vi "Facade.vi"(0 "Data In":T5, 2 "Display State In":T2, 3 "Container State":T4) -> (6 "Data Out":T5, 7 "Display State Out":T2, 8 "Action":T1)   [LabVIEW 2013, in "BarCodes.lvlib" / "Barcode.xctl"]
uses:
  Barcode.xctl
  Data.ctl
  <vilib>/_xctls/Container State.ctl
  State.ctl
  BarcodeType.ctl
  <vilib>/_xctls/Action.ctl
  EAN-13/EAN-13.lvclass
  Code39/Code39.lvclass
  Code128/Code128.lvclass
  UPC/UPC.lvclass
  Linear Barcode/Linear Barcode.lvclass
  BarCode/Write Dark Color.vi
  BarCode/Write Light Color.vi
  BarCode/Write Scale.vi
  <vilib>/_xctls/XControlSupport.lvlib
  BarCodes.lvlib
panel:
  out "Barcode":picture
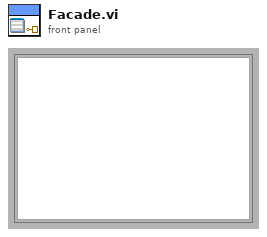
[diagram p1: front panel]
types:
  T1 = typedef "XControlSupport.lvlib/Action.ctl" = cluster{"Data Changed?":bool, "State Changed?":bool, "Action Name":string}
  T2 = typedef "BarCodes.lvlib/Barcode.xctl/State.ctl" = cluster{"BarcodeType":T3, "Scale":u8, "Dark Color":u32, "Light Color":u32}
  T3 = typedef "BarCodes.lvlib/BarcodeType.ctl" = enum16{"EAN-13", "UPC", "Code 39 (3 of 9)", "Code 128"}
  T4 = typedef "XControlSupport.lvlib/Container State.ctl" = cluster{"Indicator?":bool, "Run Mode?":bool, " Refnum":refnum<vi>}
  T5 = typedef "BarCodes.lvlib/Barcode.xctl/Data.ctl" = string
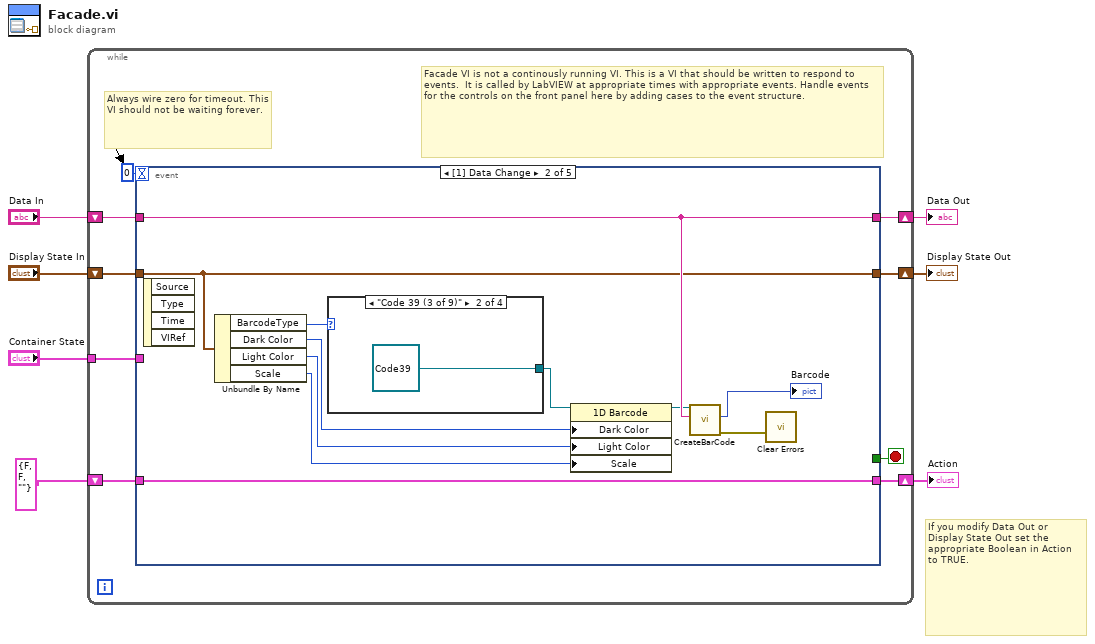
[diagram p0: block diagram]
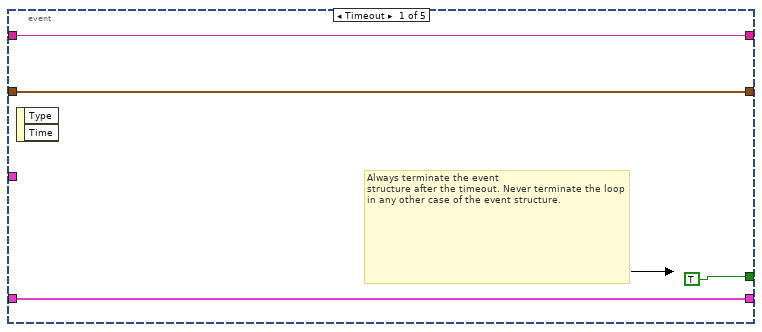
[diagram p2: hidden frame]
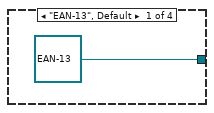
[diagram p3: hidden frame]
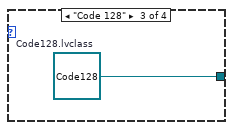
[diagram p4: hidden frame]
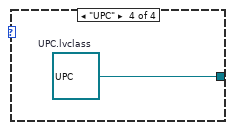
[diagram p5: hidden frame]
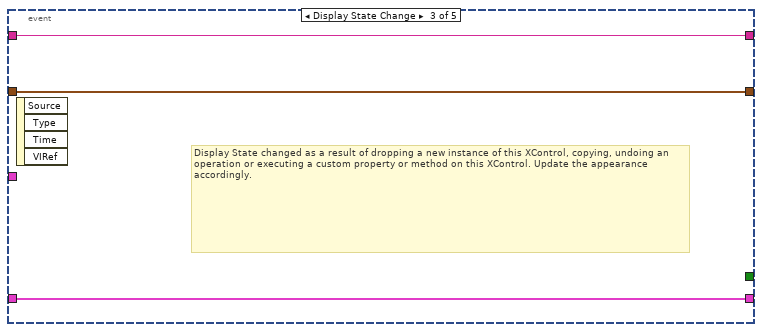
[diagram p6: hidden frame]
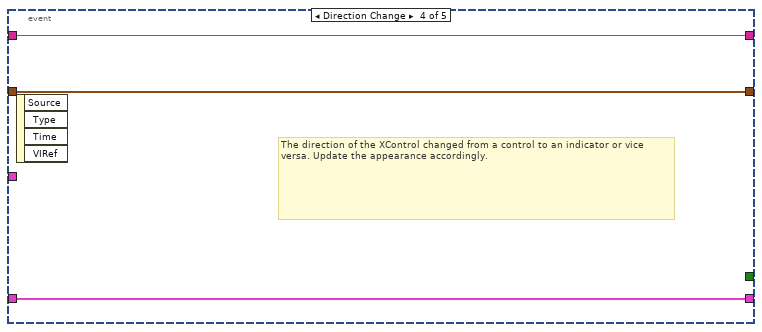
[diagram p7: hidden frame]
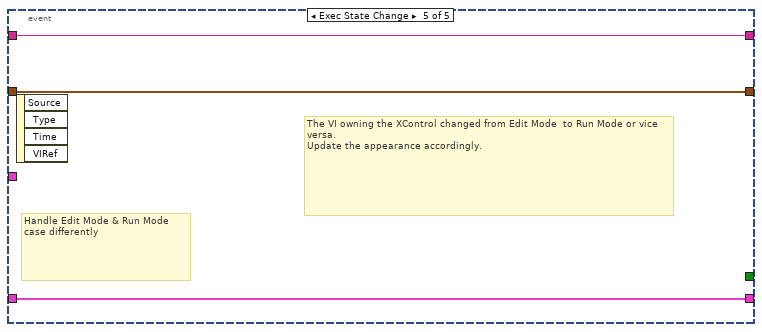
[diagram p8: hidden frame]
diagram:
  # "If you modify Data Out or\nDisplay State Out set the\nappropriate Boolean in Action\nto TRUE."
  n1 = while {
    shift-right: [w15] -> w4
    shift-left: "Display State In" -> [w16]
    tunnel: "Container State" -> [w12]
    shift-right: [w10] -> w7
    shift-left: "Data In" -> [w11]
    shift-right: [w8] -> w2
    shift-left: T1 {"Data Changed?"=FALSE, "State Changed?"=FALSE, "Action Name"=""} ("Action") -> [w9]
    stop <- w14 stop-if-true
    # "Facade VI is not a continously running VI. This is a VI that should be written to respond to events.  It is called by LabVIEW at appropriate times with appropriate events. Handle events for the controls on the front panel here by adding cases to the event structure."
    # "Always wire zero for timeout. This\nVI should not be waiting forever."
    n2 = event shown="[1] Data Change" {
      selector: _ -> [_ _ _ _ _]
      dyn-events: _ -> [_ _ _ _ _]
      timeout: 0 -> [_ _ _ _ _]
      tunnel: w16 -> [w18 w29 w38 w41 w44]
      tunnel: [w18 w29 w38 w41 w44] -> w15
      tunnel: [TRUE _ _ _ _] -> w14
      tunnel: w12 -> [_ _ _ _ _]
      tunnel: w11 -> [w17 w30 w37 w40 w43]
      tunnel: [w17 w30 w37 w40 w43] -> w10
      tunnel: [w19 w31 w36 w39 w42] -> w8
      tunnel: w9 -> [w19 w31 w36 w39 w42]
      event Timeout {
        # "Always terminate the event\nstructure after the timeout. Never terminate the loop in any other case of the event structure."
        n3 = event-data() -> ()  [unwired: 1 in, 2 out]
      }
      event Data Change {
        n4 = event-data() -> ()  [unwired: 1 in, 4 out]
        n5 = Unbundle By Name(w29) -> ("BarcodeType"=w28:T3, "Dark Color"=w24:u32, "Light Color"=w23:u32, "Scale"=w22:u8)
        n6 = case shown="\"Code 39 (3 of 9)\"" w28 {
          tunnel: [refnum<class "EAN-13.lvclass"> refnum ("EAN-13.lvclass") refnum<class "Code39.lvclass"> refnum ("Code39.lvclass") w34 w35] -> w25
          frame "EAN-13", Default {
          }
          frame "Code 39 (3 of 9)" {
          }
          frame "Code 128" {
            w34 = refnum<class "Code128.lvclass"> refnum  # Code128.lvclass
          }
          frame "UPC" {
            w35 = refnum<class "UPC.lvclass"> refnum  # UPC.lvclass
          }
        }
        n7 = property class="1D Barcode"(reference=w25, "Dark Color"=w24, "Light Color"=w23, "Scale"=w22) -> (reference out=w21:refnum<class "Linear Barcode.lvclass">)  [unwired: 1 in, 1 out]
        n8 = call-dynamic "CreateBarCode.vi"("Input"=w30, "BarCode in"=w21) -> ("error out"=w26:errorcluster, "Barcode"=→"Barcode":picture)  [unwired: 6 in, 2 out]
        n9 = call <vilib>:"Clear Errors.vi"("error in (no error)"=w26) -> ()  [unwired: 6 in, 1 out]
      }
      event Display State Change {
        # "Display State changed as a result of dropping a new instance of this XControl, copying, undoing an operation or executing a custom property or method on this XControl. Update the appearance accordingly."
        n10 = event-data() -> ()  [unwired: 1 in, 4 out]
      }
      event Direction Change {
        # "The direction of the XControl changed from a control to an indicator or vice versa. Update the appearance accordingly."
        n11 = event-data() -> ()  [unwired: 1 in, 4 out]
      }
      event Exec State Change {
        # "The VI owning the XControl changed from Edit Mode  to Run Mode or vice versa.\nUpdate the appearance accordingly."
        # "Handle Edit Mode & Run Mode\ncase differently"
        n12 = event-data() -> ()  [unwired: 1 in, 4 out]
      }
    }
  }
  "Display State Out" <- w4
  "Data Out" <- w7
  "Action" <- w2
